vi "Initialize OAuth for GitHub.vi"(5 "Allow Signup (T)":bool=TRUE, 7 "login":string, 9 "GitHub Access Scope":T2={"repo"=FALSE, "repo:status"=TRUE, "repo:invite"=FALSE, "repo_deployment"=FALSE, "public_repo"=TRUE, "admin:repo_hook"=FALSE, "write:repo_hook"=FALSE, "read:repo_hook"=FALSE, "admin:org"=FALSE, "write:org"=FALSE, "read:org"=FALSE, "admin:org_hook"=FALSE, "admin:public_key"=FALSE, "write:public_key"=FALSE, "read:public_key"=FALSE, "admin:gpg_key"=FALSE, "write:gpg_key"=FALSE, "read:gpg_key"=FALSE, "user"=FALSE, "read:user"=TRUE, "user:email"=FALSE, "user:follow"=FALSE, "gist"=FALSE, "notifications"=FALSE, "delete_repo"=FALSE, "write:discussion"=FALSE, "read:discussion"=TRUE, "write:packages"=FALSE, "read:packages"=TRUE, "delete:packages"=FALSE, "workflow"=FALSE, "security_events"=FALSE}, 10 "Client Secret":string, 11 "Client ID":string) -> (3 "Oauth2.GitHub":refnum<class "Oauth2.GitHub.lvclass">)   [LabVIEW 2017, in "Oauth2.GitHub.lvclass"]
uses:
  Oauth2.GitHub.lvclass
  D:/GitHub/Oauth2/source/Oauth2/Oauth2.lvclass
  GitHub Access Scope -- cluster.ctl
  Oauth2/OAuth2 Flow -- enum.ctl
  Oauth2/Oauth2.lvclass
  <vilib>/LabVIEW Open Source Project/Data Manipulation/Variant/OpenVariant.lvlib
panel:
  in  "Grant Flow (PKCE)":T1=enum."Authorization Code (PKCE)"
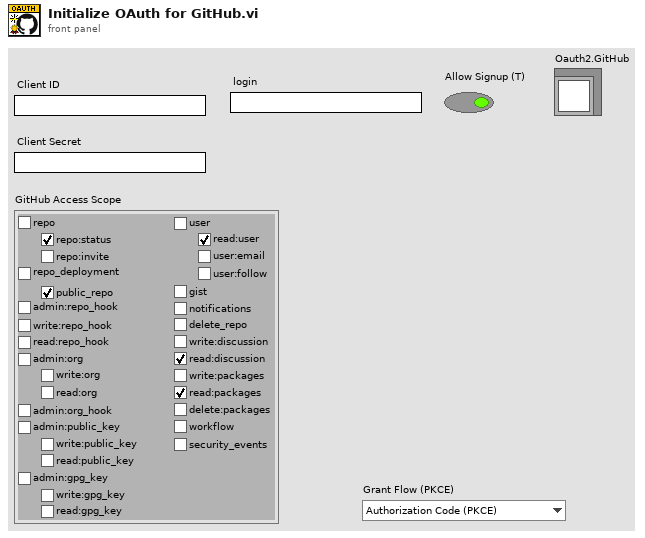
[diagram p1: front panel]
types:
  T1 = typedef "Oauth2.lvclass/OAuth2 Flow -- enum.ctl" = enum16{"Authorization Code", "Authorization Code (PKCE)", "Implicit", "Resource Owner Credentials", "Client Credentials", "Refresh Token", "Device Code"}
  T2 = typedef "Oauth2.GitHub.lvclass/GitHub Access Scope -- cluster.ctl" = cluster{"repo":bool, "repo:status":bool, "repo:invite":bool, "repo_deployment":bool, "public_repo":bool, "admin:repo_hook":bool, "write:repo_hook":bool, "read:repo_hook":bool, "admin:org":bool, "write:org":bool, "read:org":bool, "admin:org_hook":bool, "admin:public_key":bool, "write:public_key":bool, "read:public_key":bool, "admin:gpg_key":bool, "write:gpg_key":bool, "read:gpg_key":bool, "user":bool, "read:user":bool, "user:email":bool, "user:follow":bool, "gist":bool, "notifications":bool, "delete_repo":bool, "write:discussion":bool, "read:discussion":bool, "write:packages":bool, "read:packages":bool, "delete:packages":bool, "workflow":bool, "security_events":bool}
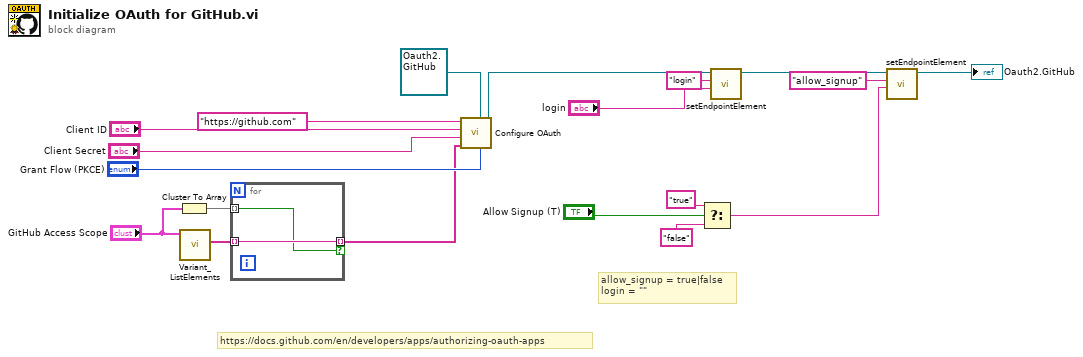
[diagram p0: block diagram]
diagram:
  # "allow_signup = true|false\t\nlogin = \"\""
  # "https://docs.github.com/en/developers/apps/authorizing-oauth-apps"
  n1 = Cluster To Array(cluster="GitHub Access Scope") -> (array=w13:bool[])
  n2 = call <vilib>:"Variant_ListElements.vi"("Variant"="GitHub Access Scope") -> ("element names"=w14:string[])  [unwired: 7 in, 3 out]
  n3 = for {
    tunnel: [w21] -> w1 mode=indexing if=w20
    tunnel: w14 -> [w21] mode=indexing
    tunnel: w13 -> [w20] mode=indexing
  }
  n4 = call "Configure OAuth.vi"("Grant Flow (PKCE)"="Grant Flow (PKCE)", "Oauth2 in"=refnum<class "Oauth2.GitHub.lvclass"> refnum ("Oauth2.GitHub in"), "scopes"=w1, "Client Secret"="Client Secret", "Client ID"="Client ID", "Authorization Server URI"="https://github.com") -> ("Oauth2"=w11:refnum<class "Oauth2.GitHub.lvclass">)  [unwired: 4 in, 1 out]
  n5 = Select(t="true" ("Endpoint Name"), s="Allow Signup (T)", f="false" ("Endpoint Name")) -> (s? t:f=w3:string)
  n6 = call "setEndpointElement.vi"("Value"="login", "Endpoint Name"="login", "Oauth2 in"=w11) -> ("Oauth2 out"=w12:refnum<class "Oauth2.GitHub.lvclass">)  [unwired: 7 in, 1 out]
  n7 = call "setEndpointElement.vi"("Value"=w3, "Endpoint Name"="allow_signup", "Oauth2 in"=w12) -> ("Oauth2 out"=→"Oauth2.GitHub":refnum<class "Oauth2.GitHub.lvclass">)  [unwired: 7 in, 1 out]
